vi "test_LoadCommandlineArgs_SuccessFile.vi"() -> (3 "Pass?":bool)   [LabVIEW 2019, in "Tests.SolutionBuilder.lvlib"]
uses:
  Tests.SolutionBuilder.lvlib
  SolutionBuilder/Community/Options.ctl
  SolutionBuilder/SolutionBuilder.lvclass
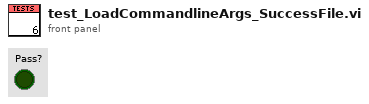
[diagram p1: front panel]
types:
  T1 = typedef "SolutionBuilder.lvlib/SolutionBuilder.lvclass/Options.ctl" = cluster{"Path":path, "Preview?":bool, "Quiet?":bool, "Log file":path, "Success file":path, "Rebuild?":bool, "Keep split projects?":bool}
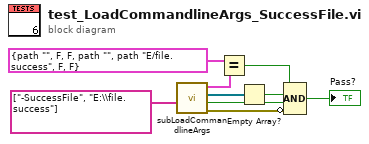
[diagram p0: block diagram]
diagram:
  n1 = call "subLoadCommandlineArgs.vi"("App.Args"=string[] ["-SuccessFile", "E:\\file.success"]) -> ("error out"=w7:errorcluster, "From command line?"=w1:bool, "Pre-built libraries"=w4:refnum<class "ProjectItem.lvclass">[], "Options"=w5:T1)  [unwired: 6 in, 1 out]
  n2 = Equal?(x=T1 {"Path"=path "", "Preview?"=FALSE, "Quiet?"=FALSE, "Log file"=path "", "Success file"=path "E:/file.success", "Rebuild?"=FALSE, "Keep split projects?"=FALSE} ("Options"), y=w5) -> (x = y?=w2:bool)
  n3 = Empty Array?(array=w4) -> (empty?=w3:bool)
  n4 = Compound Arithmetic op=AND(w2, w3, w1, invert w7) -> (→"Pass?":bool)
